vi "HRV_EEG_version3.vi"() -> ()   [LabVIEW 2014]
uses:
  <vilib>/Utility/file.llb/Read From Spreadsheet File (string).vi
panel:
  out "PPI_icon1":dbl[](graph)
  out "PPI_icon2":dbl[](graph)
  out "PPI_icon3":dbl[](graph)
  out "PPI_icon4":dbl[](graph)
  out "PPI_icon5":dbl[](graph)
  out "PPI_icon6":dbl[](graph)
  out "PPI_icon7":dbl[](graph)
  out "PPI_icon8":dbl[](graph)
  out "PPI_icon9":dbl[](graph)
  out "HF_icon1":dbl[](graph)
  out "HF_icon2":dbl[](graph)
  out "HF_icon3":dbl[](graph)
  out "HF_icon4":dbl[](graph)
  out "HF_icon5":dbl[](graph)
  out "HF_icon6":dbl[](graph)
  out "HF_icon7":dbl[](graph)
  out "HF_icon8":dbl[](graph)
  out "HF_icon9":dbl[](graph)
  out "LF_icon1":dbl[](graph)
  out "LF_icon2":dbl[](graph)
  out "LF_icon3":dbl[](graph)
  out "LF_icon4":dbl[](graph)
  out "LF_icon5":dbl[](graph)
  out "LF_icon6":dbl[](graph)
  out "LF_icon7":dbl[](graph)
  out "LF_icon8":dbl[](graph)
  out "LF_icon9":dbl[](graph)
  out "VLF_icon9":dbl[](graph)
  out "VLF_icon8":dbl[](graph)
  out "VLF_icon7":dbl[](graph)
  out "VLF_icon6":dbl[](graph)
  out "VLF_icon5":dbl[](graph)
  out "VLF_icon4":dbl[](graph)
  out "VLF_icon3":dbl[](graph)
  out "VLF_icon2":dbl[](graph)
  out "error out 6":errorcluster
  out "PPI_Path":path
  out "error out 5":errorcluster
  out "HF_Path":path
  out "error out 4":errorcluster
  out "LF_Path":path
  out "VLF_path":path
  out "ERP_Path":path
  out "error out 3":errorcluster
  out "error out 2":errorcluster
  out "error out":errorcluster
  out "ERP_target9":dbl[](graph)
  out "ERP_target8":dbl[](graph)
  out "ERP_target7":dbl[](graph)
  out "ERP_target6":dbl[](graph)
  out "ERP_target5":dbl[](graph)
  out "ERP_target4":dbl[](graph)
  out "ERP_target3":dbl[](graph)
  out "ERP_target2":dbl[](graph)
  out "ERP_target1":dbl[](graph)
  in  "피험자 이름":path=path "C:/Users/Jaehong/Desktop/안전복지프로젝트/1차 2차 실험 데이터/피험자이름.txt"
  out "VLF_icon1":dbl[](graph)
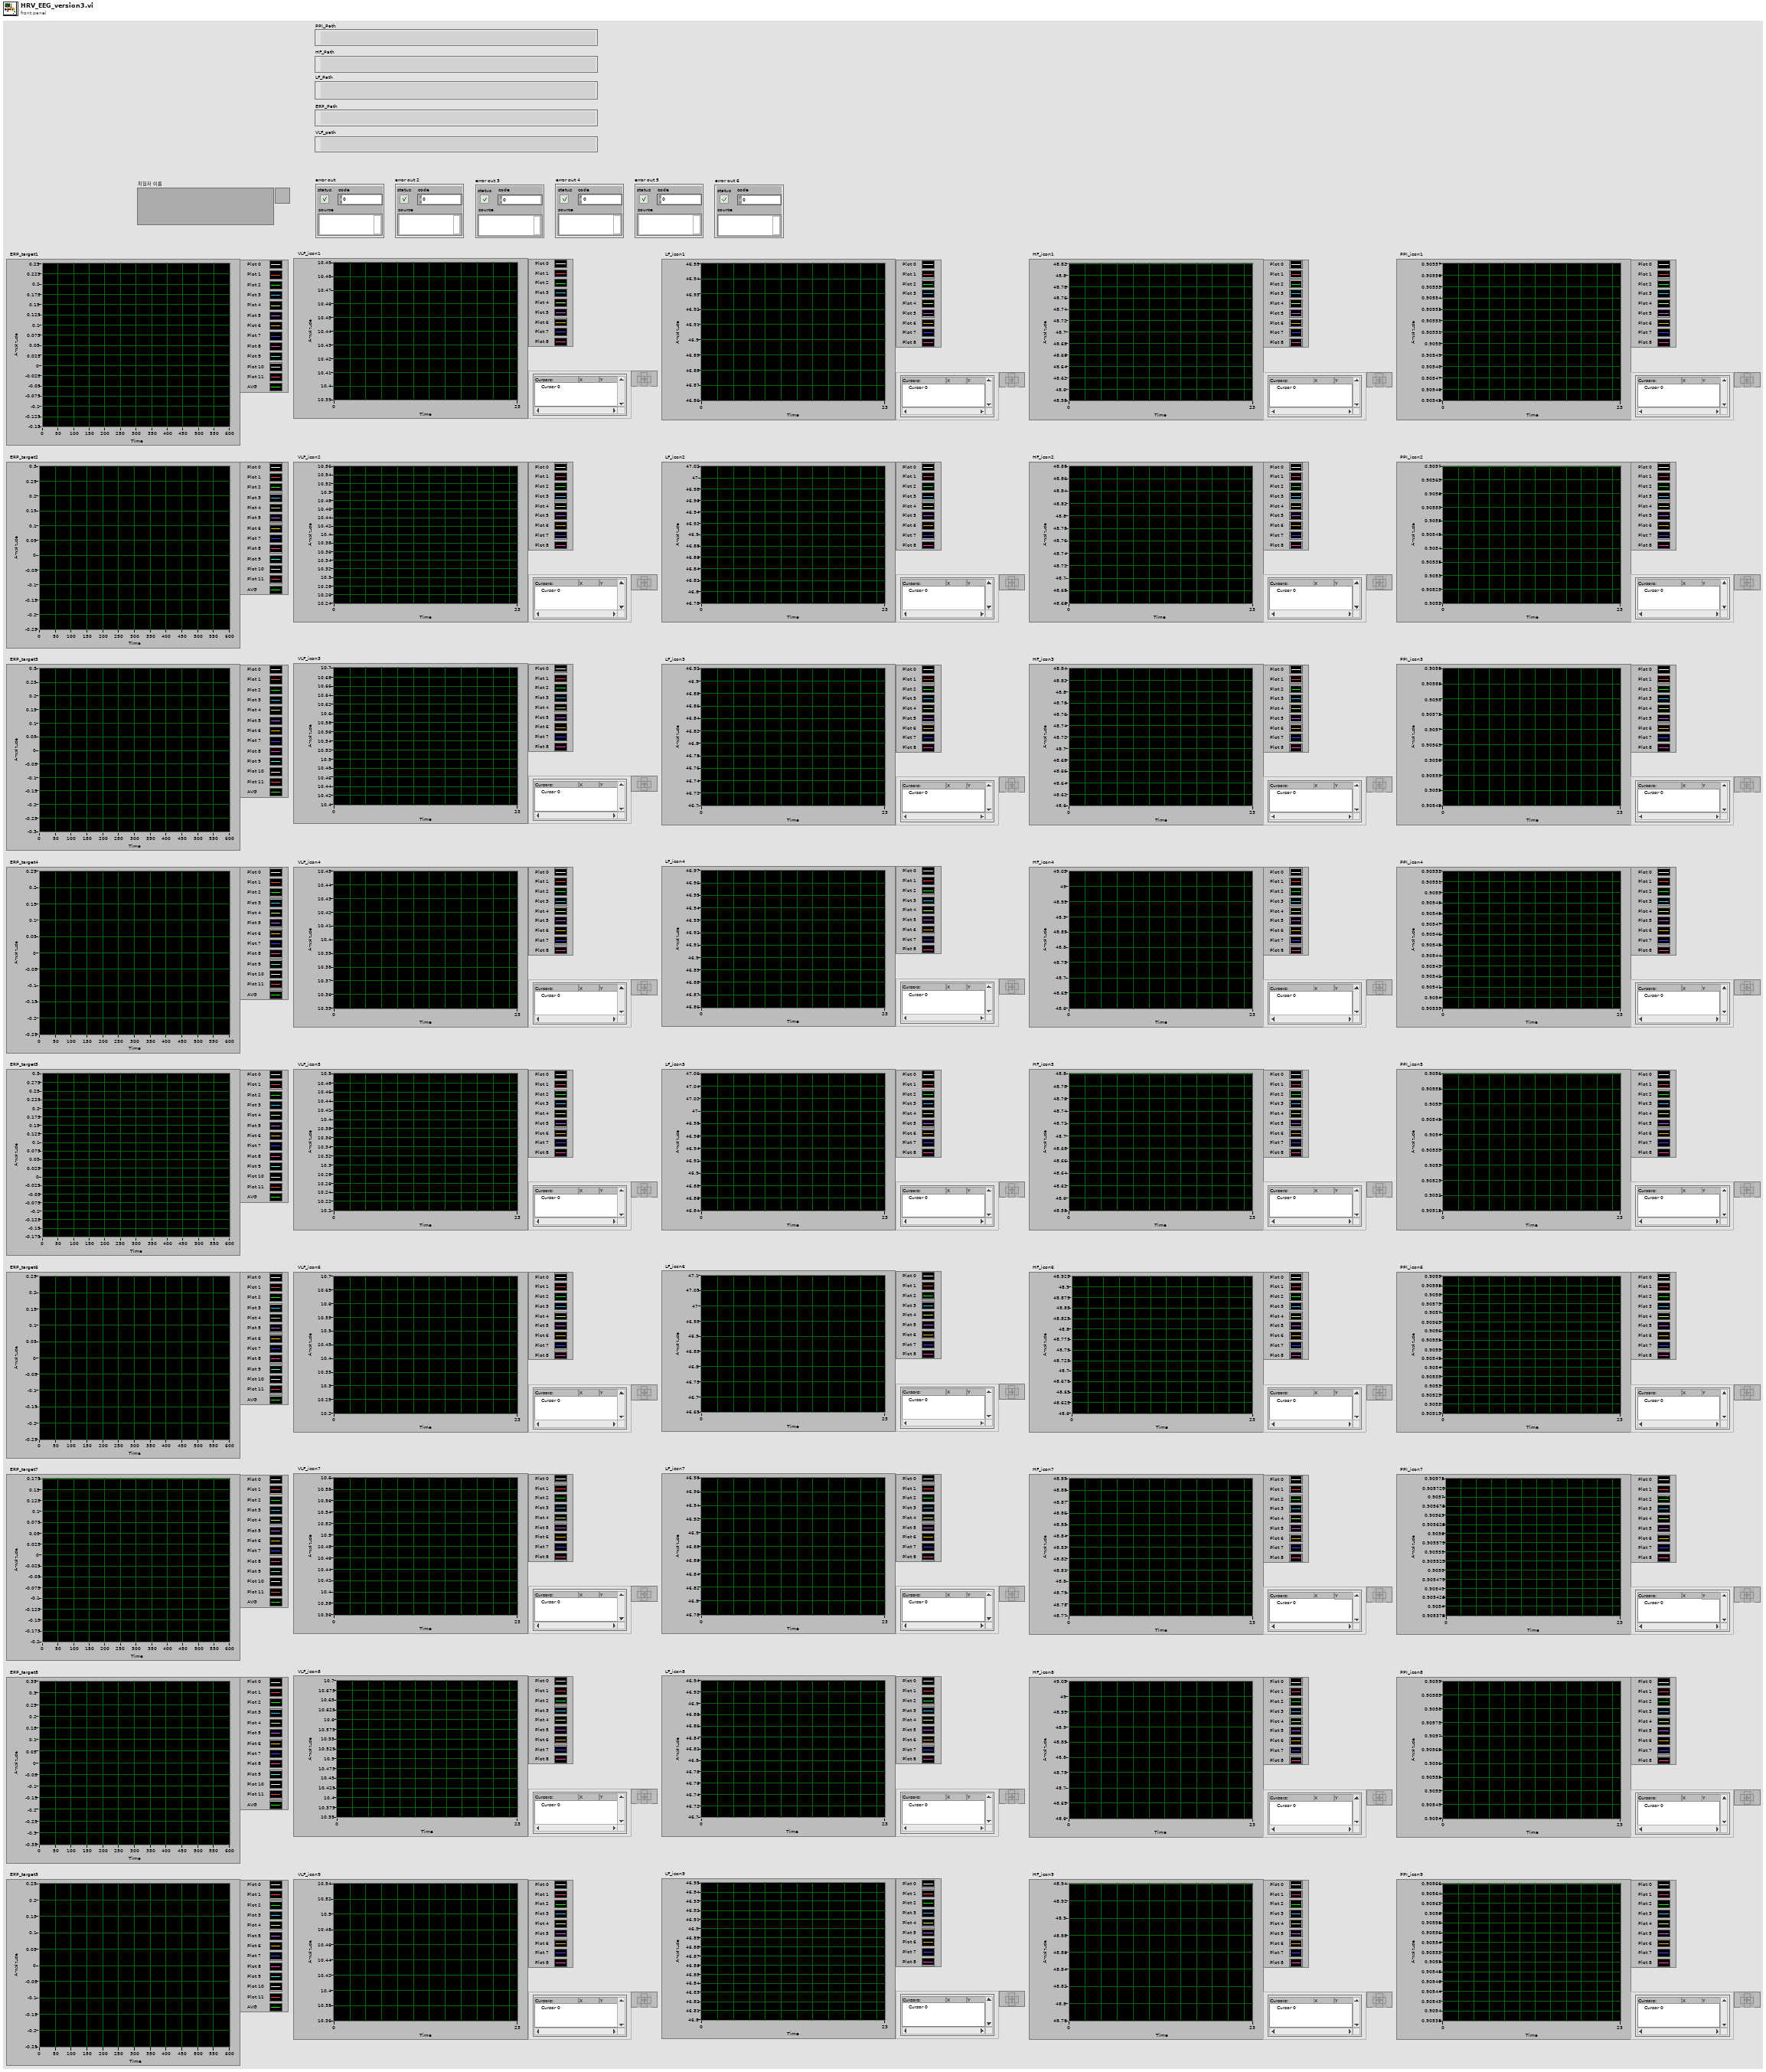
[diagram p1: front panel]
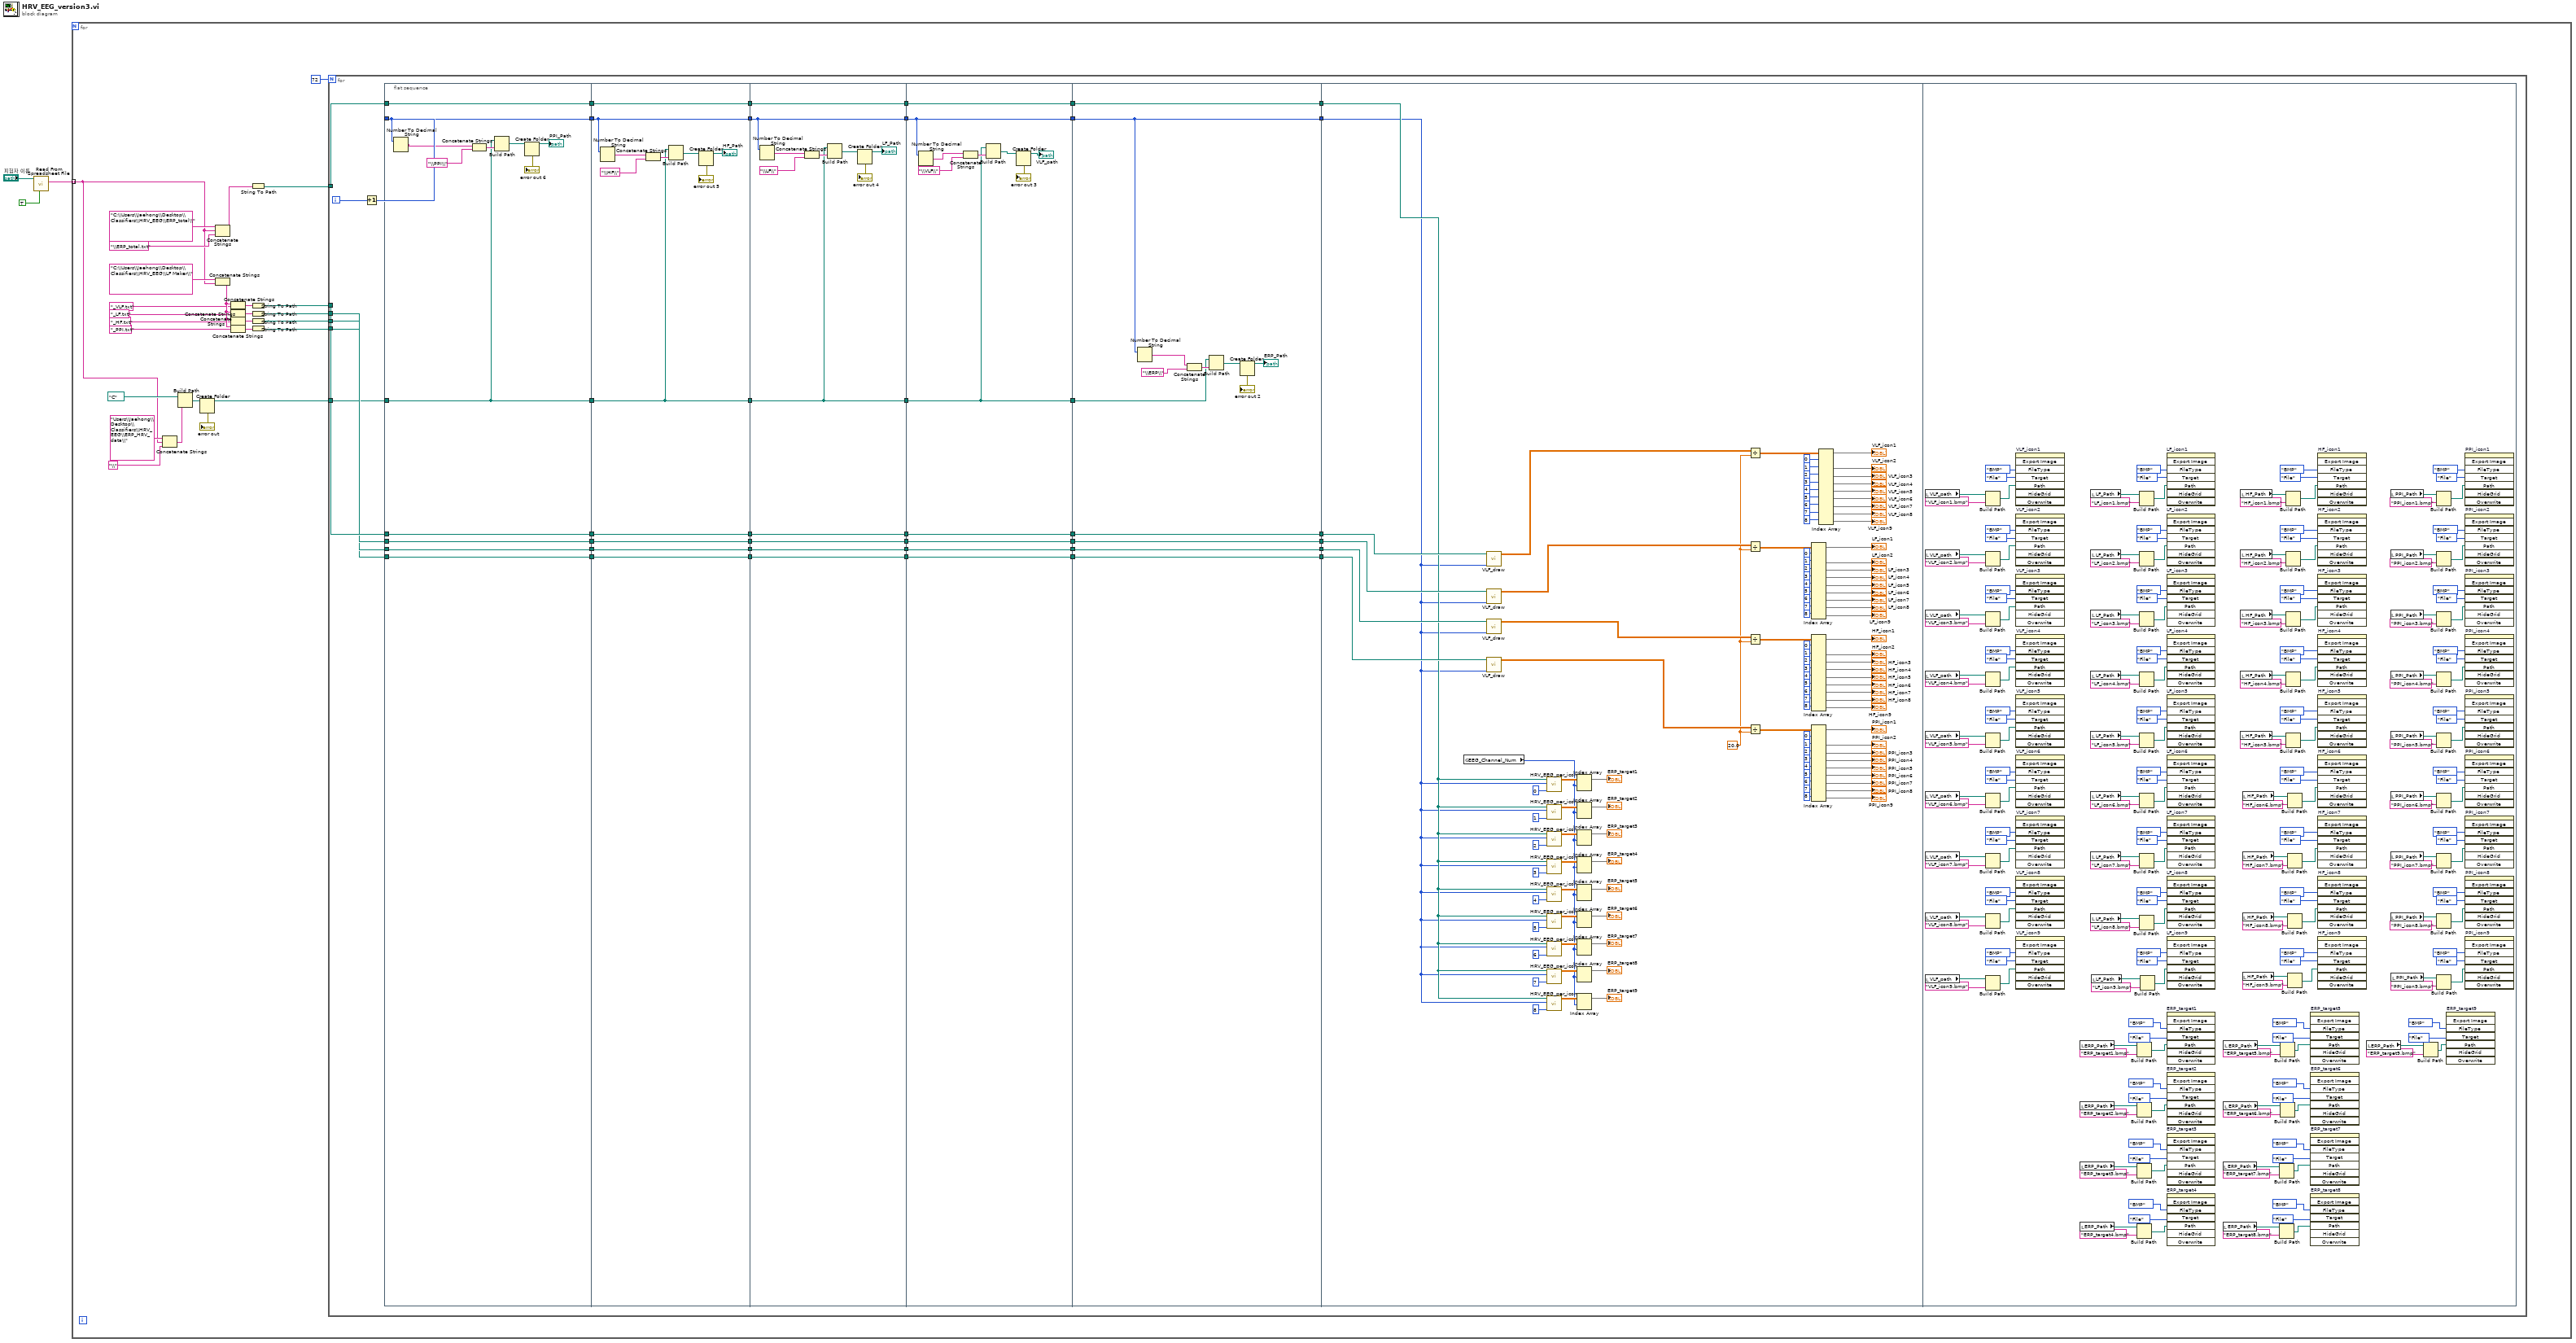
[diagram p0: block diagram]
diagram:
  n1 = call-poly <vilib>:"Read From Spreadsheet File.vi"("transpose (no:F)"=TRUE, "file path (dialog if empty)"="피험자 이름") -> ("first row"=w1:string[])  [unwired: 5 in, 4 out]
  n2 = for {
    tunnel: w1 -> [w8] mode=indexing
    n3 = Concatenate Strings("Users\\Jaehong\\Desktop\\Classifiers\\HRV_EEG\\ERP_HRV_data\\", w8, "\\") -> (w9:string)
    n4 = Build Path(base path=path "C:/", name or relative path=w9) -> (appended path=w6:path)
    n5 = Create Folder(path (use dialog)=w6) -> (created path=w4:path, error out=→"error out":errorcluster)  [unwired: 2 in, 1 out]
    n6 = Concatenate Strings("C:\\Users\\Jaehong\\Desktop\\Classifiers\\HRV_EEG\\ERP_total\\", w8, "\\ERP_total.txt") -> (w27:string)
    n7 = Concatenate Strings("C:\\Users\\Jaehong\\Desktop\\Classifiers\\HRV_EEG\\LF Maker\\", w8) -> (w24:string)
    n8 = Concatenate Strings(w24, "_VLF.txt") -> (w19:string)
    n9 = Concatenate Strings(w24, "_LF.txt") -> (w18:string)
    n10 = Concatenate Strings(w24, "_HF.txt") -> (w17:string)
    n11 = Concatenate Strings(w24, "_PPI.txt") -> (w16:string)
    n12 = String To Path(string=w27) -> (path=w26:path)
    n13 = String To Path(string=w19) -> (path=w15:path)
    n14 = String To Path(string=w18) -> (path=w14:path)
    n15 = String To Path(string=w17) -> (path=w13:path)
    n16 = String To Path(string=w16) -> (path=w12:path)
    n17 = for {
      N: 72 -> [_]
      tunnel: w26 -> [w67]
      tunnel: w15 -> [w71]
      tunnel: w14 -> [w70]
      tunnel: w13 -> [w69]
      tunnel: w12 -> [w68]
      tunnel: w4 -> [w65]
      i -> [w72]
      n18 = Increment(x=w72) -> (x+1=w66:i32)
      n19 = flat-sequence {
        tunnel: w65 -> [w73]
        tunnel: w66 -> [w80]
        tunnel: w67 -> [w81]
        tunnel: w68 -> [w82]
        tunnel: w69 -> [w83]
        tunnel: w70 -> [w84]
        tunnel: w71 -> [w85]
        tunnel: [w85] -> w58
        tunnel: [w84] -> w57
        tunnel: [w83] -> w56
        tunnel: [w82] -> w55
        tunnel: [w81] -> w54
        tunnel: [w80] -> w53
        tunnel: [w73] -> w52
        tunnel: w58 -> [w98]
        tunnel: [w98] -> w51
        tunnel: w57 -> [w97]
        tunnel: [w97] -> w50
        tunnel: w56 -> [w96]
        tunnel: [w96] -> w49
        tunnel: w55 -> [w95]
        tunnel: [w95] -> w48
        tunnel: w54 -> [w94]
        tunnel: [w94] -> w47
        tunnel: w53 -> [w86]
        tunnel: [w86] -> w46
        tunnel: w52 -> [w88]
        tunnel: [w88] -> w45
        tunnel: w51 -> [w111]
        tunnel: [w111] -> w44
        tunnel: w50 -> [w110]
        tunnel: [w110] -> w43
        tunnel: w49 -> [w109]
        tunnel: [w109] -> w42
        tunnel: w48 -> [w108]
        tunnel: [w108] -> w41
        tunnel: w47 -> [w107]
        tunnel: [w107] -> w40
        tunnel: w46 -> [w99]
        tunnel: [w99] -> w39
        tunnel: w45 -> [w101]
        tunnel: [w101] -> w38
        tunnel: w44 -> [w124]
        tunnel: [w124] -> w37
        tunnel: w43 -> [w123]
        tunnel: [w123] -> w36
        tunnel: w42 -> [w122]
        tunnel: [w122] -> w35
        tunnel: w41 -> [w121]
        tunnel: [w121] -> w34
        tunnel: w40 -> [w120]
        tunnel: [w120] -> w33
        tunnel: w39 -> [w113]
        tunnel: [w113] -> w32
        tunnel: w38 -> [w112]
        tunnel: [w112] -> w31
        tunnel: [w137] -> w64
        tunnel: [w136] -> w63
        tunnel: [w135] -> w62
        tunnel: [w134] -> w61
        tunnel: [w133] -> w60
        tunnel: [w125] -> w59
        tunnel: w31 -> [w127]
        tunnel: w32 -> [w125]
        tunnel: w33 -> [w133]
        tunnel: w34 -> [w134]
        tunnel: w35 -> [w135]
        tunnel: w36 -> [w136]
        tunnel: w37 -> [w137]
        tunnel: w64 -> [w228]
        tunnel: w63 -> [w227]
        tunnel: w62 -> [w226]
        tunnel: w61 -> [w225]
        tunnel: w60 -> [w215]
        tunnel: w59 -> [w214]
        frame #0 {
          n20 = Number To Decimal String(number=w80) -> (decimal integer string=w74:string)  [unwired: 1 in]
          n21 = Concatenate Strings(w74, "\\PPI\\") -> (w77:string)
          n22 = Build Path(base path=w73, name or relative path=w77) -> (appended path=w75:path)
          n23 = Create Folder(path (use dialog)=w75) -> (created path=→"PPI_Path":path, error out=→"error out 6":errorcluster)  [unwired: 2 in, 1 out]
        }
        frame #1 {
          n24 = Number To Decimal String(number=w86) -> (decimal integer string=w87:string)  [unwired: 1 in]
          n25 = Concatenate Strings(w87, "\\HF\\") -> (w91:string)
          n26 = Build Path(base path=w88, name or relative path=w91) -> (appended path=w93:path)
          n27 = Create Folder(path (use dialog)=w93) -> (created path=→"HF_Path":path, error out=→"error out 5":errorcluster)  [unwired: 2 in, 1 out]
        }
        frame #2 {
          n28 = Number To Decimal String(number=w99) -> (decimal integer string=w100:string)  [unwired: 1 in]
          n29 = Concatenate Strings(w100, "\\LF\\") -> (w104:string)
          n30 = Build Path(base path=w101, name or relative path=w104) -> (appended path=w102:path)
          n31 = Create Folder(path (use dialog)=w102) -> (created path=→"LF_Path":path, error out=→"error out 4":errorcluster)  [unwired: 2 in, 1 out]
        }
        frame #3 {
          n32 = Number To Decimal String(number=w113) -> (decimal integer string=w114:string)  [unwired: 1 in]
          n33 = Concatenate Strings(w114, "\\VLF\\") -> (w117:string)
          n34 = Build Path(base path=w112, name or relative path=w117) -> (appended path=w119:path)
          n35 = Create Folder(path (use dialog)=w119) -> (created path=→"VLF_path":path, error out=→"error out 3":errorcluster)  [unwired: 2 in, 1 out]
        }
        frame #4 {
          n36 = Number To Decimal String(number=w125) -> (decimal integer string=w126:string)  [unwired: 1 in]
          n37 = Concatenate Strings(w126, "\\ERP\\") -> (w130:string)
          n38 = Build Path(base path=w127, name or relative path=w130) -> (appended path=w129:path)
          n39 = Create Folder(path (use dialog)=w129) -> (created path=→"ERP_Path":path, error out=→"error out 2":errorcluster)  [unwired: 2 in, 1 out]
        }
        frame #5 {
          w238 = 20.0
          n40 = global read "Control_Panel.vi" "EEG_Channel_Num"() -> (w138:i32)
          n41 = call "VLF_draw.vi"("Trial_Number"=w214, "HRV(VLF, LF, HF, PPI)"=w228) -> ("Icon1"=w250:dbl[][])  [unwired: 9 in]
          n42 = call "VLF_draw.vi"("Trial_Number"=w214, "HRV(VLF, LF, HF, PPI)"=w227) -> ("Icon1"=w252:dbl[][])  [unwired: 9 in]
          n43 = call "VLF_draw.vi"("Trial_Number"=w214, "HRV(VLF, LF, HF, PPI)"=w226) -> ("Icon1"=w249:dbl[][])  [unwired: 9 in]
          n44 = call "VLF_draw.vi"("Trial_Number"=w214, "HRV(VLF, LF, HF, PPI)"=w225) -> ("Icon1"=w248:dbl[][])  [unwired: 9 in]
          n45 = call "HRV_EEG_per_icon.vi"("Icon Number"=0, "Trial_Number"=w214, "ERP_Total"=w215) -> ("Icon1"=w237:dbl[][])  [unwired: 8 in]
          n46 = call "HRV_EEG_per_icon.vi"("Icon Number"=1, "Trial_Number"=w214, "ERP_Total"=w215) -> ("Icon1"=w236:dbl[][])  [unwired: 8 in]
          n47 = call "HRV_EEG_per_icon.vi"("Icon Number"=2, "Trial_Number"=w214, "ERP_Total"=w215) -> ("Icon1"=w235:dbl[][])  [unwired: 8 in]
          n48 = call "HRV_EEG_per_icon.vi"("Icon Number"=3, "Trial_Number"=w214, "ERP_Total"=w215) -> ("Icon1"=w234:dbl[][])  [unwired: 8 in]
          n49 = call "HRV_EEG_per_icon.vi"("Icon Number"=4, "Trial_Number"=w214, "ERP_Total"=w215) -> ("Icon1"=w233:dbl[][])  [unwired: 8 in]
          n50 = call "HRV_EEG_per_icon.vi"("Icon Number"=5, "Trial_Number"=w214, "ERP_Total"=w215) -> ("Icon1"=w232:dbl[][])  [unwired: 8 in]
          n51 = call "HRV_EEG_per_icon.vi"("Icon Number"=6, "Trial_Number"=w214, "ERP_Total"=w215) -> ("Icon1"=w231:dbl[][])  [unwired: 8 in]
          n52 = call "HRV_EEG_per_icon.vi"("Icon Number"=7, "Trial_Number"=w214, "ERP_Total"=w215) -> ("Icon1"=w230:dbl[][])  [unwired: 8 in]
          n53 = call "HRV_EEG_per_icon.vi"("Icon Number"=8, "Trial_Number"=w214, "ERP_Total"=w215) -> ("Icon1"=w229:dbl[][])  [unwired: 8 in]
          n54 = Index Array(array=w237, index (row)=w138) -> (element=→"ERP_target1":dbl[])  [unwired: 1 in]
          n55 = Index Array(array=w236, index (row)=w138) -> (element=→"ERP_target2":dbl[])  [unwired: 1 in]
          n56 = Index Array(array=w235, index (row)=w138) -> (element=→"ERP_target3":dbl[])  [unwired: 1 in]
          n57 = Index Array(array=w234, index (row)=w138) -> (element=→"ERP_target4":dbl[])  [unwired: 1 in]
          n58 = Index Array(array=w233, index (row)=w138) -> (element=→"ERP_target5":dbl[])  [unwired: 1 in]
          n59 = Index Array(array=w232, index (row)=w138) -> (element=→"ERP_target6":dbl[])  [unwired: 1 in]
          n60 = Index Array(array=w231, index (row)=w138) -> (element=→"ERP_target7":dbl[])  [unwired: 1 in]
          n61 = Index Array(array=w230, index (row)=w138) -> (element=→"ERP_target8":dbl[])  [unwired: 1 in]
          n62 = Index Array(array=w229, index (row)=w138) -> (element=→"ERP_target9":dbl[])  [unwired: 1 in]
          n63 = Divide(x=w250, y=w238) -> (x/y=w251:dbl[][])
          n64 = Divide(x=w252, y=w238) -> (x/y=w177:dbl[][])
          n65 = Divide(x=w249, y=w238) -> (x/y=w158:dbl[][])
          n66 = Divide(x=w248, y=w238) -> (x/y=w139:dbl[][])
          n67 = Index Array(array=w177, index (row) #1=0 ("index (row)"), index (row) #2=1 ("index (row)"), index (row) #3=2 ("index (row)"), index (row) #4=3 ("index (row)"), index (row) #5=4 ("index (row)"), index (row) #6=5 ("index (row)"), index (row) #7=6 ("index (row)"), index (row) #8=7 ("index (row)"), index (row) #9=8 ("index (row)")) -> (element #1=→"LF_icon1":dbl[], element #2=→"LF_icon2":dbl[], element #3=→"LF_icon3":dbl[], element #4=→"LF_icon4":dbl[], element #5=→"LF_icon5":dbl[], element #6=→"LF_icon6":dbl[], element #7=→"LF_icon7":dbl[], element #8=→"LF_icon8":dbl[], element #9=→"LF_icon9":dbl[])  [unwired: 9 in]
          n68 = Index Array(array=w158, index (row) #1=0 ("index (row)"), index (row) #2=1 ("index (row)"), index (row) #3=2 ("index (row)"), index (row) #4=3 ("index (row)"), index (row) #5=4 ("index (row)"), index (row) #6=5 ("index (row)"), index (row) #7=6 ("index (row)"), index (row) #8=7 ("index (row)"), index (row) #9=8 ("index (row)")) -> (element #1=→"HF_icon1":dbl[], element #2=→"HF_icon2":dbl[], element #3=→"HF_icon3":dbl[], element #4=→"HF_icon4":dbl[], element #5=→"HF_icon5":dbl[], element #6=→"HF_icon6":dbl[], element #7=→"HF_icon7":dbl[], element #8=→"HF_icon8":dbl[], element #9=→"HF_icon9":dbl[])  [unwired: 9 in]
          n69 = Index Array(array=w139, index (row) #1=0 ("index (row)"), index (row) #2=1 ("index (row)"), index (row) #3=2 ("index (row)"), index (row) #4=3 ("index (row)"), index (row) #5=4 ("index (row)"), index (row) #6=5 ("index (row)"), index (row) #7=6 ("index (row)"), index (row) #8=7 ("index (row)"), index (row) #9=8 ("index (row)")) -> (element #1=→"PPI_icon1":dbl[], element #2=→"PPI_icon2":dbl[], element #3=→"PPI_icon3":dbl[], element #4=→"PPI_icon4":dbl[], element #5=→"PPI_icon5":dbl[], element #6=→"PPI_icon6":dbl[], element #7=→"PPI_icon7":dbl[], element #8=→"PPI_icon8":dbl[], element #9=→"PPI_icon9":dbl[])  [unwired: 9 in]
          n70 = Index Array(array=w251, index (row) #1=0 ("index (row)"), index (row) #2=1 ("index (row)"), index (row) #3=2 ("index (row)"), index (row) #4=3 ("index (row)"), index (row) #5=4 ("index (row)"), index (row) #6=5 ("index (row)"), index (row) #7=6 ("index (row)"), index (row) #8=7 ("index (row)"), index (row) #9=8 ("index (row)")) -> (element #1=→"VLF_icon1":dbl[], element #2=→"VLF_icon2":dbl[], element #3=→"VLF_icon3":dbl[], element #4=→"VLF_icon4":dbl[], element #5=→"VLF_icon5":dbl[], element #6=→"VLF_icon6":dbl[], element #7=→"VLF_icon7":dbl[], element #8=→"VLF_icon8":dbl[], element #9=→"VLF_icon9":dbl[])  [unwired: 9 in]
        }
        frame #6 {
          n71 = local read "VLF_path"() -> (w341:path)
          n72 = local read "VLF_path"() -> (w337:path)
          n73 = local read "VLF_path"() -> (w335:path)
          n74 = local read "VLF_path"() -> (w331:path)
          n75 = local read "VLF_path"() -> (w329:path)
          n76 = local read "VLF_path"() -> (w325:path)
          n77 = local read "VLF_path"() -> (w323:path)
          n78 = local read "VLF_path"() -> (w319:path)
          n79 = local read "VLF_path"() -> (w318:path)
          n80 = Build Path(base path=w341, name or relative path="VLF_icon1.bmp") -> (appended path=w342:path)
          n81 = Build Path(base path=w337, name or relative path="VLF_icon2.bmp") -> (appended path=w339:path)
          n82 = Build Path(base path=w335, name or relative path="VLF_icon3.bmp") -> (appended path=w336:path)
          n83 = Build Path(base path=w331, name or relative path="VLF_icon4.bmp") -> (appended path=w333:path)
          n84 = Build Path(base path=w329, name or relative path="VLF_icon5.bmp") -> (appended path=w330:path)
          n85 = Build Path(base path=w325, name or relative path="VLF_icon6.bmp") -> (appended path=w327:path)
          n86 = Build Path(base path=w323, name or relative path="VLF_icon7.bmp") -> (appended path=w324:path)
          n87 = Build Path(base path=w319, name or relative path="VLF_icon8.bmp") -> (appended path=w321:path)
          n88 = Build Path(base path=w318, name or relative path="VLF_icon9.bmp") -> (appended path=w317:path)
          n89 = invoke on="VLF_icon1" class="WFGraph (strict)" method="Export Image"("FileType"=enum32{"BMP", "EPS", "EMF", "PICT"}."BMP" ("File Type"), "Target"=enum32{"File", "Clipboard"}."File", "Path"=w342) -> ()  [unwired: 5 in, 8 out]
          n90 = invoke on="VLF_icon2" class="WFGraph (strict)" method="Export Image"("FileType"=enum32{"BMP", "EPS", "EMF", "PICT"}."BMP" ("File Type"), "Target"=enum32{"File", "Clipboard"}."File", "Path"=w339) -> ()  [unwired: 5 in, 8 out]
          n91 = invoke on="VLF_icon3" class="WFGraph (strict)" method="Export Image"("FileType"=enum32{"BMP", "EPS", "EMF", "PICT"}."BMP" ("File Type"), "Target"=enum32{"File", "Clipboard"}."File", "Path"=w336) -> ()  [unwired: 5 in, 8 out]
          n92 = invoke on="VLF_icon4" class="WFGraph (strict)" method="Export Image"("FileType"=enum32{"BMP", "EPS", "EMF", "PICT"}."BMP" ("File Type"), "Target"=enum32{"File", "Clipboard"}."File", "Path"=w333) -> ()  [unwired: 5 in, 8 out]
          n93 = invoke on="VLF_icon5" class="WFGraph (strict)" method="Export Image"("FileType"=enum32{"BMP", "EPS", "EMF", "PICT"}."BMP" ("File Type"), "Target"=enum32{"File", "Clipboard"}."File", "Path"=w330) -> ()  [unwired: 5 in, 8 out]
          n94 = invoke on="VLF_icon6" class="WFGraph (strict)" method="Export Image"("FileType"=enum32{"BMP", "EPS", "EMF", "PICT"}."BMP" ("File Type"), "Target"=enum32{"File", "Clipboard"}."File", "Path"=w327) -> ()  [unwired: 5 in, 8 out]
          n95 = invoke on="VLF_icon7" class="WFGraph (strict)" method="Export Image"("FileType"=enum32{"BMP", "EPS", "EMF", "PICT"}."BMP" ("File Type"), "Target"=enum32{"File", "Clipboard"}."File", "Path"=w324) -> ()  [unwired: 5 in, 8 out]
          n96 = invoke on="VLF_icon8" class="WFGraph (strict)" method="Export Image"("FileType"=enum32{"BMP", "EPS", "EMF", "PICT"}."BMP" ("File Type"), "Target"=enum32{"File", "Clipboard"}."File", "Path"=w321) -> ()  [unwired: 5 in, 8 out]
          n97 = invoke on="VLF_icon9" class="WFGraph (strict)" method="Export Image"("FileType"=enum32{"BMP", "EPS", "EMF", "PICT"}."BMP" ("File Type"), "Target"=enum32{"File", "Clipboard"}."File", "Path"=w317) -> ()  [unwired: 5 in, 8 out]
          n98 = local read "ERP_Path"() -> (w271:path)
          n99 = local read "ERP_Path"() -> (w275:path)
          n100 = local read "ERP_Path"() -> (w277:path)
          n101 = local read "ERP_Path"() -> (w281:path)
          n102 = local read "LF_Path"() -> (w380:path)
          n103 = local read "LF_Path"() -> (w377:path)
          n104 = local read "LF_Path"() -> (w376:path)
          n105 = local read "LF_Path"() -> (w373:path)
          n106 = local read "LF_Path"() -> (w372:path)
          n107 = local read "LF_Path"() -> (w369:path)
          n108 = local read "LF_Path"() -> (w368:path)
          n109 = local read "LF_Path"() -> (w364:path)
          n110 = local read "LF_Path"() -> (w363:path)
          n111 = Build Path(base path=w271, name or relative path="ERP_target1.bmp") -> (appended path=w273:path)
          n112 = Build Path(base path=w275, name or relative path="ERP_target2.bmp") -> (appended path=w276:path)
          n113 = Build Path(base path=w277, name or relative path="ERP_target3.bmp") -> (appended path=w279:path)
          n114 = Build Path(base path=w281, name or relative path="ERP_target4.bmp") -> (appended path=w282:path)
          n115 = Build Path(base path=w380, name or relative path="LF_icon1.bmp") -> (appended path=w387:path)
          n116 = Build Path(base path=w377, name or relative path="LF_icon2.bmp") -> (appended path=w386:path)
          n117 = Build Path(base path=w376, name or relative path="LF_icon3.bmp") -> (appended path=w384:path)
          n118 = Build Path(base path=w373, name or relative path="LF_icon4.bmp") -> (appended path=w385:path)
          n119 = Build Path(base path=w372, name or relative path="LF_icon5.bmp") -> (appended path=w383:path)
          n120 = Build Path(base path=w369, name or relative path="LF_icon6.bmp") -> (appended path=w382:path)
          n121 = Build Path(base path=w368, name or relative path="LF_icon7.bmp") -> (appended path=w381:path)
          n122 = Build Path(base path=w364, name or relative path="LF_icon8.bmp") -> (appended path=w366:path)
          n123 = Build Path(base path=w363, name or relative path="LF_icon9.bmp") -> (appended path=w362:path)
          n124 = invoke on="LF_icon1" class="WFGraph (strict)" method="Export Image"("FileType"=enum32{"BMP", "EPS", "EMF", "PICT"}."BMP" ("File Type"), "Target"=enum32{"File", "Clipboard"}."File", "Path"=w387) -> ()  [unwired: 5 in, 8 out]
          n125 = invoke on="LF_icon2" class="WFGraph (strict)" method="Export Image"("FileType"=enum32{"BMP", "EPS", "EMF", "PICT"}."BMP" ("File Type"), "Target"=enum32{"File", "Clipboard"}."File", "Path"=w386) -> ()  [unwired: 5 in, 8 out]
          n126 = invoke on="LF_icon3" class="WFGraph (strict)" method="Export Image"("FileType"=enum32{"BMP", "EPS", "EMF", "PICT"}."BMP" ("File Type"), "Target"=enum32{"File", "Clipboard"}."File", "Path"=w384) -> ()  [unwired: 5 in, 8 out]
          n127 = invoke on="LF_icon4" class="WFGraph (strict)" method="Export Image"("FileType"=enum32{"BMP", "EPS", "EMF", "PICT"}."BMP" ("File Type"), "Target"=enum32{"File", "Clipboard"}."File", "Path"=w385) -> ()  [unwired: 5 in, 8 out]
          n128 = invoke on="LF_icon5" class="WFGraph (strict)" method="Export Image"("FileType"=enum32{"BMP", "EPS", "EMF", "PICT"}."BMP" ("File Type"), "Target"=enum32{"File", "Clipboard"}."File", "Path"=w383) -> ()  [unwired: 5 in, 8 out]
          n129 = invoke on="LF_icon6" class="WFGraph (strict)" method="Export Image"("FileType"=enum32{"BMP", "EPS", "EMF", "PICT"}."BMP" ("File Type"), "Target"=enum32{"File", "Clipboard"}."File", "Path"=w382) -> ()  [unwired: 5 in, 8 out]
          n130 = invoke on="LF_icon7" class="WFGraph (strict)" method="Export Image"("FileType"=enum32{"BMP", "EPS", "EMF", "PICT"}."BMP" ("File Type"), "Target"=enum32{"File", "Clipboard"}."File", "Path"=w381) -> ()  [unwired: 5 in, 8 out]
          n131 = invoke on="LF_icon8" class="WFGraph (strict)" method="Export Image"("FileType"=enum32{"BMP", "EPS", "EMF", "PICT"}."BMP" ("File Type"), "Target"=enum32{"File", "Clipboard"}."File", "Path"=w366) -> ()  [unwired: 5 in, 8 out]
          n132 = invoke on="LF_icon9" class="WFGraph (strict)" method="Export Image"("FileType"=enum32{"BMP", "EPS", "EMF", "PICT"}."BMP" ("File Type"), "Target"=enum32{"File", "Clipboard"}."File", "Path"=w362) -> ()  [unwired: 5 in, 8 out]
          n133 = invoke on="ERP_target1" class="WFGraph (strict)" method="Export Image"("FileType"=enum32{"BMP", "EPS", "EMF", "PICT"}."BMP" ("File Type"), "Target"=enum32{"File", "Clipboard"}."File", "Path"=w273) -> ()  [unwired: 5 in, 8 out]
          n134 = invoke on="ERP_target2" class="WFGraph (strict)" method="Export Image"("FileType"=enum32{"BMP", "EPS", "EMF", "PICT"}."BMP" ("File Type"), "Target"=enum32{"File", "Clipboard"}."File", "Path"=w276) -> ()  [unwired: 5 in, 8 out]
          n135 = invoke on="ERP_target3" class="WFGraph (strict)" method="Export Image"("FileType"=enum32{"BMP", "EPS", "EMF", "PICT"}."BMP" ("File Type"), "Target"=enum32{"File", "Clipboard"}."File", "Path"=w279) -> ()  [unwired: 5 in, 8 out]
          n136 = invoke on="ERP_target4" class="WFGraph (strict)" method="Export Image"("FileType"=enum32{"BMP", "EPS", "EMF", "PICT"}."BMP" ("File Type"), "Target"=enum32{"File", "Clipboard"}."File", "Path"=w282) -> ()  [unwired: 5 in, 8 out]
          n137 = local read "ERP_Path"() -> (w288:path)
          n138 = local read "ERP_Path"() -> (w289:path)
          n139 = local read "ERP_Path"() -> (w284:path)
          n140 = local read "ERP_Path"() -> (w285:path)
          n141 = local read "HF_Path"() -> (w423:path)
          n142 = local read "HF_Path"() -> (w422:path)
          n143 = local read "HF_Path"() -> (w419:path)
          n144 = local read "HF_Path"() -> (w418:path)
          n145 = local read "HF_Path"() -> (w415:path)
          n146 = local read "HF_Path"() -> (w414:path)
          n147 = local read "HF_Path"() -> (w411:path)
          n148 = local read "HF_Path"() -> (w410:path)
          n149 = local read "HF_Path"() -> (w406:path)
          n150 = Build Path(base path=w288, name or relative path="ERP_target7.bmp") -> (appended path=w293:path)
          n151 = Build Path(base path=w289, name or relative path="ERP_target8.bmp") -> (appended path=w294:path)
          n152 = Build Path(base path=w284, name or relative path="ERP_target5.bmp") -> (appended path=w291:path)
          n153 = Build Path(base path=w285, name or relative path="ERP_target6.bmp") -> (appended path=w292:path)
          n154 = Build Path(base path=w423, name or relative path="HF_icon1.bmp") -> (appended path=w432:path)
          n155 = Build Path(base path=w422, name or relative path="HF_icon2.bmp") -> (appended path=w431:path)
          n156 = Build Path(base path=w419, name or relative path="HF_icon3.bmp") -> (appended path=w430:path)
          n157 = Build Path(base path=w418, name or relative path="HF_icon4.bmp") -> (appended path=w429:path)
          n158 = Build Path(base path=w415, name or relative path="HF_icon5.bmp") -> (appended path=w428:path)
          n159 = Build Path(base path=w414, name or relative path="HF_icon6.bmp") -> (appended path=w427:path)
          n160 = Build Path(base path=w411, name or relative path="HF_icon7.bmp") -> (appended path=w426:path)
          n161 = Build Path(base path=w410, name or relative path="HF_icon8.bmp") -> (appended path=w425:path)
          n162 = Build Path(base path=w406, name or relative path="HF_icon9.bmp") -> (appended path=w408:path)
          n163 = invoke on="ERP_target5" class="WFGraph (strict)" method="Export Image"("FileType"=enum32{"BMP", "EPS", "EMF", "PICT"}."BMP" ("File Type"), "Target"=enum32{"File", "Clipboard"}."File", "Path"=w291) -> ()  [unwired: 5 in, 8 out]
          n164 = invoke on="ERP_target6" class="WFGraph (strict)" method="Export Image"("FileType"=enum32{"BMP", "EPS", "EMF", "PICT"}."BMP" ("File Type"), "Target"=enum32{"File", "Clipboard"}."File", "Path"=w292) -> ()  [unwired: 5 in, 8 out]
          n165 = invoke on="ERP_target7" class="WFGraph (strict)" method="Export Image"("FileType"=enum32{"BMP", "EPS", "EMF", "PICT"}."BMP" ("File Type"), "Target"=enum32{"File", "Clipboard"}."File", "Path"=w293) -> ()  [unwired: 5 in, 8 out]
          n166 = invoke on="ERP_target8" class="WFGraph (strict)" method="Export Image"("FileType"=enum32{"BMP", "EPS", "EMF", "PICT"}."BMP" ("File Type"), "Target"=enum32{"File", "Clipboard"}."File", "Path"=w294) -> ()  [unwired: 5 in, 8 out]
          n167 = invoke on="HF_icon1" class="WFGraph (strict)" method="Export Image"("FileType"=enum32{"BMP", "EPS", "EMF", "PICT"}."BMP" ("File Type"), "Target"=enum32{"File", "Clipboard"}."File", "Path"=w432) -> ()  [unwired: 5 in, 8 out]
          n168 = invoke on="HF_icon2" class="WFGraph (strict)" method="Export Image"("FileType"=enum32{"BMP", "EPS", "EMF", "PICT"}."BMP" ("File Type"), "Target"=enum32{"File", "Clipboard"}."File", "Path"=w431) -> ()  [unwired: 5 in, 8 out]
          n169 = invoke on="HF_icon3" class="WFGraph (strict)" method="Export Image"("FileType"=enum32{"BMP", "EPS", "EMF", "PICT"}."BMP" ("File Type"), "Target"=enum32{"File", "Clipboard"}."File", "Path"=w430) -> ()  [unwired: 5 in, 8 out]
          n170 = invoke on="HF_icon4" class="WFGraph (strict)" method="Export Image"("FileType"=enum32{"BMP", "EPS", "EMF", "PICT"}."BMP" ("File Type"), "Target"=enum32{"File", "Clipboard"}."File", "Path"=w429) -> ()  [unwired: 5 in, 8 out]
          n171 = invoke on="HF_icon5" class="WFGraph (strict)" method="Export Image"("FileType"=enum32{"BMP", "EPS", "EMF", "PICT"}."BMP" ("File Type"), "Target"=enum32{"File", "Clipboard"}."File", "Path"=w428) -> ()  [unwired: 5 in, 8 out]
          n172 = invoke on="HF_icon6" class="WFGraph (strict)" method="Export Image"("FileType"=enum32{"BMP", "EPS", "EMF", "PICT"}."BMP" ("File Type"), "Target"=enum32{"File", "Clipboard"}."File", "Path"=w427) -> ()  [unwired: 5 in, 8 out]
          n173 = invoke on="HF_icon7" class="WFGraph (strict)" method="Export Image"("FileType"=enum32{"BMP", "EPS", "EMF", "PICT"}."BMP" ("File Type"), "Target"=enum32{"File", "Clipboard"}."File", "Path"=w426) -> ()  [unwired: 5 in, 8 out]
          n174 = invoke on="HF_icon8" class="WFGraph (strict)" method="Export Image"("FileType"=enum32{"BMP", "EPS", "EMF", "PICT"}."BMP" ("File Type"), "Target"=enum32{"File", "Clipboard"}."File", "Path"=w425) -> ()  [unwired: 5 in, 8 out]
          n175 = invoke on="HF_icon9" class="WFGraph (strict)" method="Export Image"("FileType"=enum32{"BMP", "EPS", "EMF", "PICT"}."BMP" ("File Type"), "Target"=enum32{"File", "Clipboard"}."File", "Path"=w408) -> ()  [unwired: 5 in, 8 out]
          n176 = local read "ERP_Path"() -> (w295:path)
          n177 = local read "PPI_Path"() -> (w469:path)
          n178 = local read "PPI_Path"() -> (w466:path)
          n179 = local read "PPI_Path"() -> (w465:path)
          n180 = local read "PPI_Path"() -> (w462:path)
          n181 = local read "PPI_Path"() -> (w461:path)
          n182 = local read "PPI_Path"() -> (w458:path)
          n183 = local read "PPI_Path"() -> (w457:path)
          n184 = local read "PPI_Path"() -> (w454:path)
          n185 = local read "PPI_Path"() -> (w452:path)
          n186 = Build Path(base path=w295, name or relative path="ERP_target9.bmp") -> (appended path=w297:path)
          n187 = Build Path(base path=w469, name or relative path="PPI_icon1.bmp") -> (appended path=w477:path)
          n188 = Build Path(base path=w466, name or relative path="PPI_icon2.bmp") -> (appended path=w476:path)
          n189 = Build Path(base path=w465, name or relative path="PPI_icon3.bmp") -> (appended path=w475:path)
          n190 = Build Path(base path=w462, name or relative path="PPI_icon4.bmp") -> (appended path=w474:path)
          n191 = Build Path(base path=w461, name or relative path="PPI_icon5.bmp") -> (appended path=w473:path)
          n192 = Build Path(base path=w458, name or relative path="PPI_icon6.bmp") -> (appended path=w472:path)
          n193 = Build Path(base path=w457, name or relative path="PPI_icon7.bmp") -> (appended path=w471:path)
          n194 = Build Path(base path=w454, name or relative path="PPI_icon8.bmp") -> (appended path=w470:path)
          n195 = Build Path(base path=w452, name or relative path="PPI_icon9.bmp") -> (appended path=w453:path)
          n196 = invoke on="ERP_target9" class="WFGraph (strict)" method="Export Image"("FileType"=enum32{"BMP", "EPS", "EMF", "PICT"}."BMP" ("File Type"), "Target"=enum32{"File", "Clipboard"}."File", "Path"=w297) -> ()  [unwired: 5 in, 8 out]
          n197 = invoke on="PPI_icon1" class="WFGraph (strict)" method="Export Image"("FileType"=enum32{"BMP", "EPS", "EMF", "PICT"}."BMP" ("File Type"), "Target"=enum32{"File", "Clipboard"}."File", "Path"=w477) -> ()  [unwired: 5 in, 8 out]
          n198 = invoke on="PPI_icon2" class="WFGraph (strict)" method="Export Image"("FileType"=enum32{"BMP", "EPS", "EMF", "PICT"}."BMP" ("File Type"), "Target"=enum32{"File", "Clipboard"}."File", "Path"=w476) -> ()  [unwired: 5 in, 8 out]
          n199 = invoke on="PPI_icon3" class="WFGraph (strict)" method="Export Image"("FileType"=enum32{"BMP", "EPS", "EMF", "PICT"}."BMP" ("File Type"), "Target"=enum32{"File", "Clipboard"}."File", "Path"=w475) -> ()  [unwired: 5 in, 8 out]
          n200 = invoke on="PPI_icon4" class="WFGraph (strict)" method="Export Image"("FileType"=enum32{"BMP", "EPS", "EMF", "PICT"}."BMP" ("File Type"), "Target"=enum32{"File", "Clipboard"}."File", "Path"=w474) -> ()  [unwired: 5 in, 8 out]
          n201 = invoke on="PPI_icon5" class="WFGraph (strict)" method="Export Image"("FileType"=enum32{"BMP", "EPS", "EMF", "PICT"}."BMP" ("File Type"), "Target"=enum32{"File", "Clipboard"}."File", "Path"=w473) -> ()  [unwired: 5 in, 8 out]
          n202 = invoke on="PPI_icon6" class="WFGraph (strict)" method="Export Image"("FileType"=enum32{"BMP", "EPS", "EMF", "PICT"}."BMP" ("File Type"), "Target"=enum32{"File", "Clipboard"}."File", "Path"=w472) -> ()  [unwired: 5 in, 8 out]
          n203 = invoke on="PPI_icon7" class="WFGraph (strict)" method="Export Image"("FileType"=enum32{"BMP", "EPS", "EMF", "PICT"}."BMP" ("File Type"), "Target"=enum32{"File", "Clipboard"}."File", "Path"=w471) -> ()  [unwired: 5 in, 8 out]
          n204 = invoke on="PPI_icon8" class="WFGraph (strict)" method="Export Image"("FileType"=enum32{"BMP", "EPS", "EMF", "PICT"}."BMP" ("File Type"), "Target"=enum32{"File", "Clipboard"}."File", "Path"=w470) -> ()  [unwired: 5 in, 8 out]
          n205 = invoke on="PPI_icon9" class="WFGraph (strict)" method="Export Image"("FileType"=enum32{"BMP", "EPS", "EMF", "PICT"}."BMP" ("File Type"), "Target"=enum32{"File", "Clipboard"}."File", "Path"=w453) -> ()  [unwired: 5 in, 8 out]
        }
      }
    }
  }
